vi "DalesMess Analog Read Pin Example.vi"() -> ()   [LabVIEW 2010]
doc: "An example that reads a user selectable analog input pin on the Arduino."
uses:
  <vilib>/LabVIEW Interface for Arduino/LabVIEW Interface for Arduino.lvlib
panel:
  in  "disREG":bool
  in  "enREG":bool
  in  "relPROG":bool
  in  "enPROG":bool
  in  "3V6 Off":bool
  in  "iSenseREF":bool
  in  "iSenseDUT":bool
  in  "Set Function":bool
  in  "Select Function":T1(ring)
  in  "Stop":bool
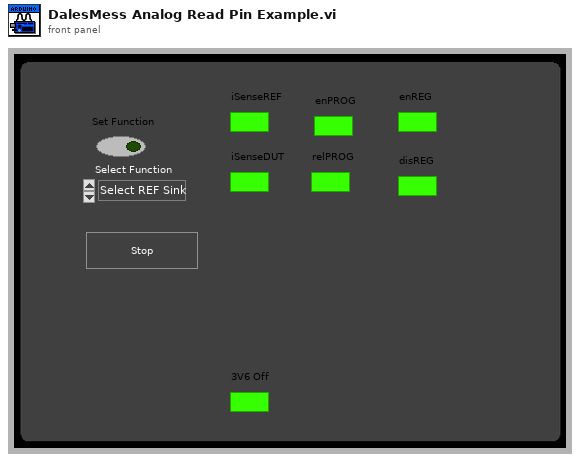
[diagram p1: front panel]
types:
  T1 = enum8{"Select REF Sink", "SelectDUT Sink", "Read AN3", "Enable PROG", "Disable PROG", "Enable Register", "Disable Register"}
  T2 = typedef "LabVIEW Interface for Arduino.lvlib/Arduino Resource.ctl" = cluster{"VISA resource":refnum<visa-resource-name>, "Board Type":T3, "Connection Type":enum8{"USB / Serial"}, "Bytes Per Packet (15)":u8}
  T3 = typedef "LabVIEW Interface for Arduino.lvlib/Board Type.ctl" = enum16{"Uno", "Dimuelanove w/Atmega 328", "Mega 2560"}
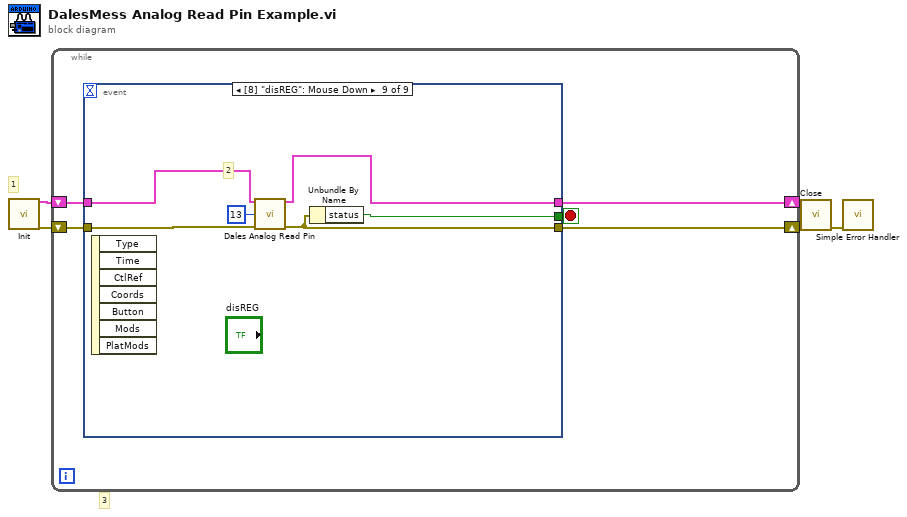
[diagram p0: block diagram]
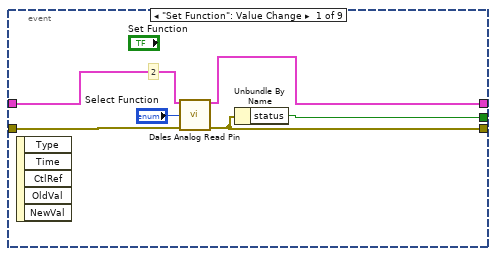
[diagram p2: hidden frame]
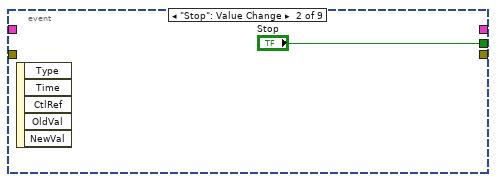
[diagram p3: hidden frame]
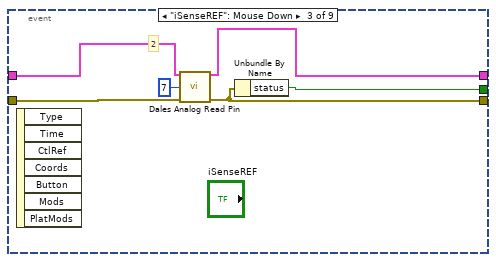
[diagram p4: hidden frame]
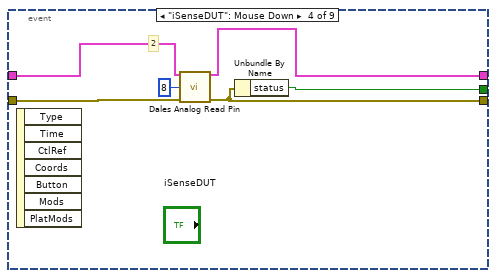
[diagram p5: hidden frame]
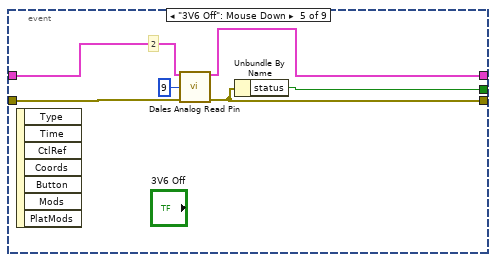
[diagram p6: hidden frame]
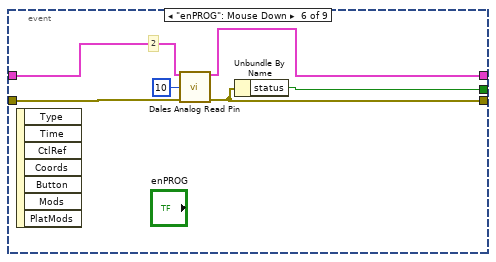
[diagram p7: hidden frame]
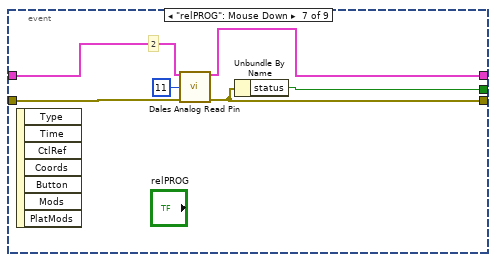
[diagram p8: hidden frame]
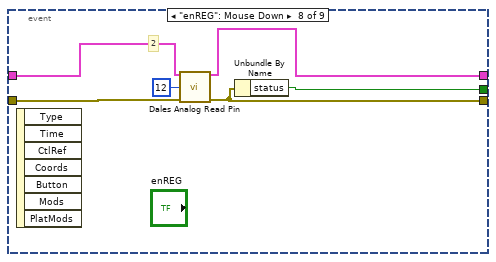
[diagram p9: hidden frame]
diagram:
  # "3"
  # "1"
  n1 = call <vilib>:"Init.vi"() -> ("Arduino Resource"=w5:T2, "error out"=w2:errorcluster)  [unwired: 18 in]
  n2 = while {
    shift-right: [w10] -> w4
    shift-left: w5 -> [w7]
    shift-right: [w9] -> w3
    shift-left: w2 -> [w6]
    stop <- w8 stop-if-true
    n3 = event shown="[8] \"disREG\": Mouse Down" {
      selector: _ -> [_ _ _ _ _ _ _ _ _]
      dyn-events: _ -> [_ _ _ _ _ _ _ _ _]
      timeout: _ -> [_ _ _ _ _ _ _ _ _]
      tunnel: [w16 _ w23 w29 w35 w41 w47 w53 w59] -> w10
      tunnel: [w15 _ w22 w28 w34 w40 w46 w52 w58] -> w9
      tunnel: [w11 "Stop" w19 w25 w31 w37 w43 w49 w55] -> w8
      tunnel: w7 -> [w14 _ w21 w27 w33 w39 w45 w51 w57]
      tunnel: w6 -> [w13 _ w20 w26 w32 w38 w44 w50 w56]
      event "Set Function": Value Change {
        # "2"
        n4 = event-data() -> ()  [unwired: 1 in, 5 out]
        n5 = call "Dales Analog Read Pin.vi"("Arduino Resource"=w14, "Analog Input Pin (0)"="Select Function", "error in"=w13) -> ("Arduino Resource"=w16:T2, "error out"=w15:errorcluster)  [unwired: 11 in]
        n6 = Unbundle By Name(w15) -> ("status"=w11:bool)
      }
      event "Stop": Value Change {
        n7 = event-data() -> ()  [unwired: 1 in, 5 out]
      }
      event "iSenseREF": Mouse Down {
        # "2"
        n8 = event-data() -> ()  [unwired: 1 in, 7 out]
        n9 = call "Dales Analog Read Pin.vi"("Arduino Resource"=w21, "Analog Input Pin (0)"=u8 7, "error in"=w20) -> ("Arduino Resource"=w23:T2, "error out"=w22:errorcluster)  [unwired: 11 in]
        n10 = Unbundle By Name(w22) -> ("status"=w19:bool)
      }
      event "iSenseDUT": Mouse Down {
        # "2"
        n11 = event-data() -> ()  [unwired: 1 in, 7 out]
        n12 = call "Dales Analog Read Pin.vi"("Arduino Resource"=w27, "Analog Input Pin (0)"=u8 8, "error in"=w26) -> ("Arduino Resource"=w29:T2, "error out"=w28:errorcluster)  [unwired: 11 in]
        n13 = Unbundle By Name(w28) -> ("status"=w25:bool)
      }
      event "3V6 Off": Mouse Down {
        # "2"
        n14 = event-data() -> ()  [unwired: 1 in, 7 out]
        n15 = call "Dales Analog Read Pin.vi"("Arduino Resource"=w33, "Analog Input Pin (0)"=u8 9, "error in"=w32) -> ("Arduino Resource"=w35:T2, "error out"=w34:errorcluster)  [unwired: 11 in]
        n16 = Unbundle By Name(w34) -> ("status"=w31:bool)
      }
      event "enPROG": Mouse Down {
        # "2"
        n17 = event-data() -> ()  [unwired: 1 in, 7 out]
        n18 = call "Dales Analog Read Pin.vi"("Arduino Resource"=w39, "Analog Input Pin (0)"=u8 10, "error in"=w38) -> ("Arduino Resource"=w41:T2, "error out"=w40:errorcluster)  [unwired: 11 in]
        n19 = Unbundle By Name(w40) -> ("status"=w37:bool)
      }
      event "relPROG": Mouse Down {
        # "2"
        n20 = event-data() -> ()  [unwired: 1 in, 7 out]
        n21 = call "Dales Analog Read Pin.vi"("Arduino Resource"=w45, "Analog Input Pin (0)"=u8 11, "error in"=w44) -> ("Arduino Resource"=w47:T2, "error out"=w46:errorcluster)  [unwired: 11 in]
        n22 = Unbundle By Name(w46) -> ("status"=w43:bool)
      }
      event "enREG": Mouse Down {
        # "2"
        n23 = event-data() -> ()  [unwired: 1 in, 7 out]
        n24 = call "Dales Analog Read Pin.vi"("Arduino Resource"=w51, "Analog Input Pin (0)"=u8 12, "error in"=w50) -> ("Arduino Resource"=w53:T2, "error out"=w52:errorcluster)  [unwired: 11 in]
        n25 = Unbundle By Name(w52) -> ("status"=w49:bool)
      }
      event "disREG": Mouse Down {
        # "2"
        n26 = event-data() -> ()  [unwired: 1 in, 7 out]
        n27 = call "Dales Analog Read Pin.vi"("Arduino Resource"=w57, "Analog Input Pin (0)"=u8 13, "error in"=w56) -> ("Arduino Resource"=w59:T2, "error out"=w58:errorcluster)  [unwired: 11 in]
        n28 = Unbundle By Name(w58) -> ("status"=w55:bool)
      }
    }
  }
  n29 = call <vilib>:"Close.vi"("Arduino Resource"=w4, "error in"=w3) -> ("error out"=w1:errorcluster)  [unwired: 13 in]
  n30 = call <vilib>:"Simple Error Handler.vi"("error in (no error)"=w1) -> ()  [unwired: 4 in, 5 out]
